vi "Main_15A.vi"() -> ()   [LabVIEW 2024]
uses:
  Utility/Universal Utility/TypeDefs_Utility/Cluster_Row-Column.ctl
  Utility/Universal Utility/TypeDefs_Utility/ENUM_4 Directions U-D-L-R.ctl
  b5234449-2328-4583-8824-3fa0b55a92a1.vi
  <vilib>/Utility/error.llb/Trim Whitespace.vi
  <vilib>/Utility/error.llb/Trim Whitespace One-Sided.vi
panel:
  out "Direction":T1
  out "Grid End":string[][](array[string])
  out "Array 2":T1[](array[typedef])
  out "Start Position":T2
  out "Grid Start":string[][](array[string])
  in  "Example 1":string="########\n#..O.O.#\n##@.O..#\n#...O..#\n#.#.O..#\n#...O..#\n#......#\n########\n\n<^^>>>vv<v>>v<<"
  in  "Use Puzzle":bool
  out "Answer 1436690":u32
  in  "Puzzle":string="##################################################\n#.......#....O....O......O..O#.OOOO....#.OO......#\n#..O.O..#O..#O..#O.OO......O....O..O....#O.......#\n#...O......O...O...O.......#O#.O.#OO.O........O.O#\n#..O..#O..#.O....OO..OO.....#.OO.....#.O#OOOOO.O.#\n#........O#.....O..OO......#.O..O#...O.O..O......#\n##O..O.O...#O.#...#O...#O..##......#............O#\n#.OO#O.O..O...O#..OO...#..###O....OO.#.O.##....#.#\n#.O...........O.....O..O.OO.O.O...O..OO....OO....#\n#OO..........O...O........O..##O.OOO.O..O..O..#.O#\n#.#O.....O.OO....#O..O...O.....O...........OO..#O#\n##.....O.......O.O.O....O.O...#O.O..O##....OO#...#\n#.OO......O.......O..#...O......#.OOOO.OOO...#O..#\n#.........O.O....OO..##.....OO...#....O.OO..OO...#\n#O....O..O..#...OOO...OOO#..OO......OO..O....OO.O#\n#....O.........O....#.#.O..OO......O.O..#O.O#OO..#\n#...O.OOO.O.O..O.........O.OO....OO.O.....OO..OOO#\n#..O.........#...OO.O#.O....OOO......O..........O#\n#........O.O.O.O..OOOOO.#.O.OO#OO.....#...O.O.#O.#\n#OO...O.#O.OOO....O....O.#.O.OOO.O..O......OOOO.O#\n#...#OO.O..O...O.OOO.....O.O.OO.#..O#...O..OO....#\n#O.OOOO.O........#O.##......#....#...OO..O.O.OO..#\n#.OOO.O.O#OO...O.O...O.........O........O..O#OOO.#\n#.#..O........#......O......O.....O....O.#..O....#\n#...#.....O.O.OOO.OO.O.O@O.O.O.O..#O....#.#.OO..O#\n#O.......#O...#O....O.#.....OO.#O.O..O.O......O..#\n#......O...OO.OO..O#....OOO.#.#....O.O....OO....O#\n#...O.O.#..OO#.O.OO...O.#.#..#O..#...##..O.......#\n##O...O..OO.O..O.OOO..O.........O#O...#..#.O..O#O#\n#O.O....#OO..OOO.#O..#O..O.#...#.#..O....O.O....##\n#.O.OOO.O....O...#O.O...OOO..O.....O.O..O.O..O..O#\n#......O...O..OO.O........O..........O....#....OO#\n#.O..OO.O.OOO..OO...........O........O.O....OO.O##\n#.O.OO#....#.........#..O...OO...OO..OO..........#\n#...OO...OO..OO.O...O.....#...O.#.....OO.O.O.O#O.#\n#OO......#...OO......O..O.O...O...#.....O......OO#\n#O...O.....O...O.O.O....O##OO.O..#..O....O#OO...O#\n#.O.O#OO..##.#O...O#O..O.O#..O...OO...OOO.......##\n#...O.#.O.#......OO.......O.OO..#.OOOOO...OO..O.##\n#............O..O.....#O.##.O.O.#....O#.......O.O#\n#.O..##..O....#O.O..#....O...OOO#.#...#..O...O...#\n#.O.OOOO..#.........O.O#....O....OO.OO.....##OOO.#\n#..O#...OO..O...O#...#..OO.OO...#....O........O.O#\n#.O.O..O....O...O.O.OO#...OO..O.OO.O.O..O...O....#\n#.O#..OO...#.OO...........OO.....OO#O.#..O.O...#.#\n#..................O.......O...OO..O..O.O.O.O##..#\n#.##.#..OO.#..........O#...O.O.O...##..O......O.O#\n#OO.O........####.......O.......O......O...##....#\n#.O........O..O..#...O.OO...#....#.#.....OO...O.##\n##################################################\n\n<><v>^vv<^<v<>^>^^<^^>>^>><vv^>^>^<v<>>^^>>v^>^<v><v><v>>^<^<<^^>^>^<<v^<<^^v><<><v>v^>^^<v<<<>v<>^>^^^><v<><v^<><vv^v>^>^>><^<vv<^>^<^<<<<<^<^vv><v>^v^^><<>>v<v>vvv^<>v<>v><<<v^<^<^vv<^v<>v<<<<<>v<^<<<^<^v^<^>^>>vv>>^^<>^^<^v<^v<<vv<vvv^<^^<>v^^><^^^v^>^>^^<<<^<v<^<><v^<^v^<>>v><^^v^vv><vv>^v>>^vv>v><v<>>>^>>^v>v^^<vv^<v>vv<^<>^>>^v^v><^v^>>^>^<<<<<><v<v<vvv><><^^v^^^<>v<>vv>v^>>>^<>>^^^><v<^<>v<^>^<vvv^>^>vvv>>v<>v<>v<><><<^vv>^<^<<>^^<v<^^>v^v<v<>>^^><>^>>>^v^<>^^^<>><v><>v><>v>^<>vvv>>><><v<><>v^vv^>v^^>>v<^<^<v^>>>^^>>v<<<v^vvvv>^^v>^v<^>^vv^v^v<^^>v>^vv<<v^^^v^<v<^v^<v><v>^^v<^^><^^<^vvv<v<<><>v^<>><<<^vv<^^<<>^^<^<^>^<><v><^>v>><><v^vv<<>>^^>vvv^><<^v<<^>^<^<<><^<>^<>vv>><v>^^<v<v>v^v^^<<>^>>^^v>>v>^^>^<><^>v<vvv>^>v<><vv<><^v>>^<^^<<<<<>^vv<<<v>^<><^<v>v^<v<v<v^<v^<>^v<vv^vv>v^^>v^>^^<v^<<v>^^v>v><<<<<^vv><v>>v><^^^v<^^vvv^^>^^^>vv<>v^<>><><<><^>^^^v^<v>>>v<>vv>vvvv^>>v<<<^vv>>>^v^v><<^vvv^<<>v<><^v><>^v>>v>^^<<>v^vvv><^^<>>^<<<<>>^>>v^^<>>>>vv>v<v^>^<^v>v>>^^>v^^v<^vv><^<^^<vv\n<<^<><v<^vvv<<vv<vv<><v^v><>><<v^<>^>>^>>^^^<^^v<vvv^v>v<>^>><^v>^^vvv^<>>>v>>vvv><^^v>vvv<vv<><v>>vv^^<>^^<^>v^<v>vv^<><v<^<>^vv>^^><>^>^v^<vvv><>^>><^<^>v>v>><v<<vv^^^>^v^vvv>>vv^^<^^<>>v<<vvv^<^<^>>v>>v<<v^<^v><v^><^>v^<v<vvvvv>>>^^v><<^^>v><<<^^<<<^><^<<^v<>^<>v<<<v>v<v<<<^v^^^<v<^^^<^<vv<>>^<^<>v^>>v^v><^vvv>^>>v><<^<<v>v>v>^v<v^<v^^v>^>>^<v^v<>^v><<>>>>>^>^<v<v>>^^v<><><<v>vv><^<>><v>>>v^v<>^><v^v^><<v<^^<vvv<v>^>vvv<>^>>v>^v<^^^v>v>v<>>^<><^<^<<v^<^>vv^v^>v^^^^^v^v><>v<><<<v^vv^>v<v<><>>^^<^<v<>^><>v^^>^^><>v>v^^>v<>>^>^^<v<^^^<<^^>^^>vv<^<^><>^^^v^^^>>^>>v<<^v^^v^<^^^v<^^>>^>^<v<>>^^>><vvv>v<v<>^<vv<v^v>^<v>v>v<>v<v<<<><<<^>>>^>^v>vv>>v^vv^<vv>><<>>v^>^^>>^v>^^v^v^<^<v><><v>v><^^^>^><v>vv<><<^^^<v<^^vv<><v<v>vv^^><><^v^<^v>v<<v>>v<vvv<<^<<v<vvv>>vv<<^<vv><>>v><vv<<>v<vv^><><^v<^<><<>>v<>v^v^<v<><v>^>v>v^vv>v<<v^>>><<<v<^v<v^^v^^>v^v>vvv>v<^v<^<<^>v>><<<v<>>vv>v><vvvvv>vv>v^<^^^<v<v^v<<v^v<^^>>v<vvv<>v>>^<v>^<v^<>^^>>^>vv^<>v^v^<vv^<>>v^^^v^^^^>^v><v<>^>v<v><>>><><^v><^^v<>v^v^>\nvv^^>v^^v<v<vvv<v<<v^>vv<>>>^v^>v>^><>v^><><v^^<^>v><vv>>><v<>v<<<^v<<>^^<vvvv^^>v>v<^>v^^<<vv^v>v^><><><<vvv>v>vv^<<<vv^<v<^>v^<^>vv<>>>vv>^^^^>vv>v^^v<>^^^>v><>>v<>v>>v<^<<>^>><^v<<^<^>><>vv>^><>^^^^^^>^<^<v<<^<<v<v^v>^vvv^<>^v^>><<<^^>^^<v>v^v<^>>><^^<v^<vv><<vvv<<^>v^^>v>v<v^v>v<^v>>v^>^<<v><v>^>^<v<><^>><>>^><^<<^v><^<<>v>><>v<<v<><^v>><^<vv>>v^<><>>^^<<v>>>v^>^v>v>^<v<>><v>^<v<v^^^>^>^vv^<vv<<<>><>><^<v<<<v>>v>^>^>v<><><^v<>><>vvv>^><<^^^<vv<vv><>vv>v^>vv>v><><<^vv>^vvvv<<<<v<v^<>>v>v><v^><v<<v>>^v^^v>^v<<v^^>v>><v<<v<^v<v^^<<<v^^<<v^>^^^^^^<><^>v^><><v^<^^<>>v^<v^v^^^<v^>^^v>v<>^><v>^^><^>^>v>>^<>vv<v<^^v<^^>v^^<>^<^>>>^<^v<vvvv>^<v^>v<<^^^<v<>^v<<<>>^<<^vv>>vvv>v<<>><>^^><vv><<<^v>>><<<vv<v><<v>^v^vv<v>^>>v<<v>v>>><v>><^^v^v^v<<>^>v^>><v^>>v><<vvv^<^vv^v>>^^>v^v<<<>^>v^^v<<vv>v^>v<<^^<<>>v<<v<v^>>^><>^vv^><^>v<<v><<<v<^vvv^v^^v^>><v>vv<>^>v^<<v><><v<^v>v>vv^^v^^<<>>^<v><>v^>>>v<^<vvv<<v<>v>v<v>vvvv>^v>v>^^>v>^><v<^>v><<>><v^vvv<^^v>v^^^^>^<v<>>^>v^<^<>^^>>><v^v>>^><^v^vv>^<v>v<\nv<^^vv><>><<^v^<^v^>^^<^>vv<<^vvvvvv^<><<vv>^<^v>>>><^v<<^<>><>><>>>><<^>>v>>^>^^>^><^<<v^v>v^v>^<^v^<>vv^v>><>vv>><>^<<v><v^v>v>>^^^<<^v><v<v^^>>^vv^>^^>^^v^<<<^>^>^><>v<<<v^>^^^>v<>^<v^v<>>><<<v<>^>v<^^<>^^v<^v>>^>><v<v>>^><^v<^<><>v>v>>>^<<><^^^<<<vvv<^>>^><^><v^<v<v><^v^v<<<><v<vv><<^v<v<<v^^<^<^^^>v^^>v><>^v^><^>>>v>><^v^v>v^<<>v^v<<^<<vv^^<v^^v<>^>^>^<>v>^v<>v>>v>vv^vv>^><><v<^<><<<>>><<>^>^<v<>>>^^<>>^>v^><^vv><^<^>>v>vv<^<v<><^v<^>>><^v<^><v><v^v^<<^><^<><^^<^v^^v>vv^^<v<<>^>>^^v^^<vv<<^vv<vv^<>vv>^>^<v^><><<><<><^v>^^v^><<<v<^<vvv>^><<>>><<v><>vv^^>>^^><<v><^<v>vv^^<^<^^^>^<v<>^v^>v^^v^<>v^<v^v<v><^>v^^><<<>^^^<<v^v<<<<>>v<v^^v^vv^vv^v>v>>^>>^vv^v^<<^vv^<v^v^<>^<^<v>v^<<v<<>^^>><v^>v^^>v^>>>v><<>><v^^^<><><v<<v<<^v>v^>><v<>^vv>^><v<^v>^<>v<<><>>v^v^>^>v>><^<^^><v><^>vv>v<vv^><^^v>^^>v^v<>v<v^^^<<><v>^^vv>v<^>vv^^v^v>>^vv^<><^<^<<<v<>><>>^>^^^^><^v<<<>v^<^^vv><^v>v^vvv><>v>^<<^^^v^^<>>v<^^v<^^^>>^vv<v^^<vvv<^<<^>v^<>^^^<^v^^<v>^><^>^^^v^^>^<>>^v^>vv<v>^<vv^^><^v^^^>v<^v<<>v<^<v\n<^><vv^v^>>^<>>>v><^vv<v^<^vv<<>v^>v<v^^^^>vv^><<v>^^^v<v^<<v<v><^^v>^<v<<^>^^^>v>v<^^>v^v><<vvv^^^>vv^v>^<vvv<vv><<>>>v>v<vv<><<><^v>vv><<^^^vv<><^<<^>^><<>^<v>^>^v<<>>v^<^vvv<v^>>v<<^>^>v<<<^v<><><^^<>^<^<v><<vv<>>^<v^^><^^v<<><vv><^>^^>v^vv^^<>^vv>v^>v>^v>v>^>^>^>><>v<^v>><^<>^v<>vv<^v<^v^<>^<>^<^^v><v^<vv>v<^>>v>>v^v^<^vvv>><v<vvv><<^^<^v<^<vvvvvv<v^^^>^^vv^^v>>>>>^^>v^>^><^><>>^<>v^>v<<<^v><v<v^^vv^<^^v>^v^<vvvv^^<^<^<<<v^v^^<v<<v><^<v><vv<^^>v<vv<^<^v<^>^^^vv^<>^<v>^v^<><>><v>v^<<><^^^>>vv<v^^<v>>^<<>v<vv>^<<v<^<<vv^^<v<vvv>^vv<v^><vv<><v>>^^>v>^<>>^^<v<v<v^<vv>><<^><v<v^<<vv^^^<v><<^<v<<<v>^<vv^><<<^^v<^>vv<>>^>^v^<v>^^v>>v^>>v>vv><<v<<v>v^vv^>vvv^^v<>^>^v><vv>^><v>v^>^v^^><>v<^<v>^<<^vv>^v<<><vv>v^>vv<>>^>>>><<^v<v>^<><v<<<<>>^v>v><^v^^>^<<<v<v^^v^<>v><^>^>^^^v><<<^>v><^><<^vvv<vv^v>v^><<><^>^<<vv^>v><>v>v<>v<vv<>v<<^v>^>^v>^^v<>v>v<<v^v>>>vv>>v>>><^^^v^>>vvv^^vv><^v^<vv^><<^v<vvv<^^v<<vv<<v<><vvv<><<>v<v>^><<>><v<v<>^<v<>vv<<><<v^>^^^^^><<><^v^v<^>v<^^^><<<^<^v><^v<>^>>v^v^<^^\n>vvv^<<>vv>vv<^^vvv>vvvv^<^>v^<vv^^v>^v<<^<<v<<vv>^v^v<<><v<><<>>><><v><<>v<<>>v<<<^>><v<v<>>>>vv>>>>^v<>^><v>>^><v<>^v^v<>^v<^v>^v^^v^^v<><^v<<>^<>><v><^<^<<<><^v^vv<<<<>>>^vv<<><<v^^vv<>vv^>v<^v^>vv<>vv<<v^<>^<<<>^><v<vv><>^v>vv^><<^^<v<<v><>^>>v><>^>vv^^>>^^<^>^^<^vv^^<>><v<<^><<v^^^<v^v<<>>>>^v^<v^>>^><<v^<v^^>>v<<<v>>>^<v^^>v^v<>^>>>>>^^^>v>v>>vv<v^^>>^v>v^^vv<<vvv<<>^^v<<>>>^<><<<>v<>>^v^><<>^>v<>^^^>v>vv<vv>^<^^v<^^>v<^^^^<<<v>><<vv<v>v^>>><v^v>v^^^v<<<v^><>><^<^<^>><>^^v>v>v>>v<>>>v^^><^v<^>><v><v^<^<^>^^^>>>v^<>^>^v^v<vvv<^^^<>><<v<<>><^v>v^v<>>vvv<vv<<><v<>^<<^vv<^vv><>v<^v><^<>>>^<v<vvv<^vv<^vv><^v^><<<v^^<<^v^v>^>v^^^^v<>^^^<<><<vv<<^>vvvv^vv>^<vv<^^<^>^<^^^>v>v^<<>^>^<<v><>^v^^^><<><>v><<<><>v^>v>^<<<>v^>^<<^vv>>>^vvv<>>vv<vvv^<v<>>>v^vvv^v>^>>v<v^>><v^<^<^<^v<vv>v>^><><><^v>>v<^^^v>^vvv^^>>^<^<^^><<>^^<v<<^>^>^>v><>v<<v><<>><^v<>v>^<>^v^>v>^<>^>^>v^<v^><<>><<>v<^v>^<<<<<<v><<>><>><>><^v^^^vv<v^v<vv>v>vv<v^^^v^><v^^v<>v><<>v>>><<v><^<><>^v<v<><<<><>>^<v^<v<v<v^v<v<><v^<>vv\n<<<v^>v>>^>v>v<v<>^^><<^^><^^vvv>>>^>^><<^^<v<><v<<>^^^^vv<^<v^><<v>>><<<<<<<vv<<><v<<<>v<v<<^vv^<v>^^^^^^><^vvv<>v^>^^vv<vv><^>><v<>><>^<<vv^^<>^>^><v><v>v<^v<v<^^^^><^<^^><^v^^<vv^<><<^>^v<v^^v^^<>><<v<^^^<>vv<^^vv^><v><<v^v>>vv^><v<^^^v<<v<<<>vv>>><v<vv>^<^<v<v<>^>v><^>v>v<^<>v^^>>^^<>^<^<v>><<^<<^^^v<v<^<^<<v<v>>^<>><^v^v^<>vv>><v^^><v>><^<^>>^^<<v^<<<>v<^<v^v<v><<^v<vv<v<<>^v^v<<><v^><>><^v^vv^>>v^^v^^^<v><<<v>>^v^><^<v<<>>>^v>^^v<><vv<^^<>^^<<v<<v<<v^^^<^v^<<>vv><<<vv^^<^^vv<^v>^<v>^^^vv^<>v<<>^vv<<vv^^<>v<><^^<vv<<v^<<^<^vv>><^>><>><v^<<v><>^<<^vvv^>v^^>v>v^^^^^^^^v^^^v^<^^^v^^vv^>>v>v^^<v><><<^>v>><^>^v^><^^v>v^vv<v^>^>^<<^^^vvvv<<>><>v<>vv<vvv<<v^^v^^vv><<>^<^>^^^^^vv>^><^^^<<><>^^v^>^^>>v^^^<^<><>^<<>>v^<v<^v<>>>^<vv>^v^>^<<>^v<<v><^v^>><>^<><<v<>><v<>^>^vvv^^>v^>>v>>^>vvvvvv>>v>^vvvv>>^^^<<v>^^^<vvv<<v<v^v^^v<><<<v^v<><<vv<<<<vvv^^^<^>v^v^v^^>^v>^<>^v>>><^vv>vv<^^^vv<>^<><><>vv^v>v>v>>>^v^<^<>^<v<v<v><^<<>^^<^<>^v>>^v^>v^>v^>v<v^>^<>v^<^<^<vvv<v<vv^v<<>>^<^v<^^^<<<^>^^>^<<v>\n^v<v^<^^>>^v><v<><^<><><>v^<>^><>v<<vvv<><>v<><<^^vv>>^^^><^^<>^>><<^^>v><v><^>^>^>><>v^<><><^^^v<^<v^<>v>vv>v>^<><<><^^<^^v<><^<<v^<<^>^^>>>^>>^^^^<^v><><<<^^<^v>v^<^v^><v>^^^><^>^vvv>^v<>v<v><<<^v>^<v<<>^^^<^>^^^<^<v<<>>>>v^>^v^>v^v<v<<^<^^<v^^>v<><^<><^>v^v><<v<v>^vv<^vv><v<v<^><>^v^<<^>vv<^^v<^vv<>>v>>^<>^>>^>>>>^v^<>><v^>vv^^>^v^>^<<<v>^><<>>>><<>^v<<>>>>>^>^^^>>><^>>v^vv^^v><vv>^v^vv^vvv^>^>v>v^vv>^v^^<vvv>vv>><<<<^<<<><>v^v^^^<>^v^<>><<^^^<>vv<<<v>v<<<^>><>^<><v<v>v<v<vv^vv<v^vv^^<<<<vv<>vv^vv<v<<v<v><><>^^><^>^<><^v^>>^<^>>>vv^><<><<^>><v<<v^v<>^v^^v^<><v>^v^^vvv<<v^v<<^^^^^<vvv<><^<>^v<<>><v^v^>>>v^^<^>v<><vv><<<<^<v<v<<<^>v<<<v^v<<^v>^^><<<v>vv<<>v<>v^v<^<>^>>><^v><>^^v><<>vv^v<^v><vvv<<vv<><^>>>v<v><<^^<v>^vv^^>^v<<^<>v^v<v><<>^vv><<<vv^v<>^<v^v<^v>^<<<>^>^vv^><>v^<>v<>>>^vv<vv^<^v^<v><>>v><vv<v>><^v^^^^>>v^>^>v^^<<^^v>vvvvv<>^vv^<^<>^<>v>>vv>v>v<>^><>v^^^vv^>v^<>^vvv<>>>v<<vv<<v>>v>><<^vvv^>v^<<v<v<<>^<><^v<<^>>>v^<^>v<<<<v>^^^^^v><>v>vv<>>^<v^^^v<>v<<>v^<>>v><^^^v^^^>^^>v>\n<>^^<<vvvvv^>vv>>>^<>^v^vv<v^<^v>^^><^>><<^^vv>v<v><v^<^<^>><><<<>v^v>vv<v^v^v>><><v>>^<v^<><v<^^^v<v<<v<<^>^v<^^>^^^vv^><>>^<<<<v<^^<v^<<^^<v>>v^^vvvv^vv>v>>vv<^^>v^vv<>v<v<v<^<v>v^>v^>>^<v><<<<<^^<>>^v^<<v^><v><>vv<v>^^<^<><v<^v<^^vv^<><v>^<<^<>^^^^^>^vv>v>^>>vv>v<>v^^<><^^>^>><>^^v>v><v<^<<<^v<>^>^v^^v>v>>^>^vv><^>^>^<><^^v><v<^>v>vv^v>^v^>^>^v<v>>v>>v^<<v^>v^>v^>>v<^<<<><>^vv<>>v<^^^>v><<<><<<vvv<v<>v<^vv^v<v><^^vvv>^^vv^<>>v>^vv^^<^<>><<>v^v^^^^^<v>v^^<<^^<^v>>>^>^^^^v>^^v><^v^>^v>^^^<>^<<^v^v>v><^^v>^vvv<<>>^v^^>^>^v<v^>>>^v><v<>vv^v>v>v^v<^v>vv>>^>v^<^^^^>^<^>v^^>>^<>^^><v>vv<^>^^<^><<>>^>^v>>v>^<^v<<vvvv^vv<>>v<><^v^v>^v^^v^v<v><<^^v><^>^>^v<vv^^^^<^^v^v<v>^><<<v><<<>^v^>v>vv<^<><^^<>^<>>vv<v<<>^><^^^^v>v<>>v<<>vv^>^vv><<vvv><>v><^v^><vvv>vv<v^<>>^v^^<<<<>>><v<>>^^><^><v<^^<<<<^^^>vv^>^v<<v<vvvv<>^^v>^>v^^><<^<^v><v>^^^>v^<>>^>vv>><^^><^^^>^>><^<>>>>vv><><^<>>v<>v>^v^>^>^><v^^>v>>>^v^vv>v>><>v^^^>><v><>v<>v^^^vv<<vv<vv><><<^<<<>vv<vv>v>^^<v>>v^>>v><<v>^^<><>^>v^<>^vvv>^<^v<<vv<\nv><^^>v>v>^<^<^<<v^<<v><^^<<<^^>><<<^>^^vv<^>vvv<>^^^<<>^vv^v>^^v>^v^^v^<>^vvvv^>vvv>^^<<v>v>^>vvv>><<<v>>v^><>>^<<v^<^^v>><<^^^^><v^<<^^>^^v>^vv^>vvv>v^v^vv^>>^<^<>>v<v^v><<^^^><^^vv^v>v>^>v<v>^><>^<>^>^>vvv>>^<^>^vv>^^<>^^>^><^>^<v<>>^vvv<vv^v>>><<<v^>^v^><^v^<v>vv<<<><<<vv^^vv>>v<v<>v<><^^vv<>>>^v^^<^<<>^<<^<vv^<v>>>v^<>^>>vv>>>^^v^v<vv<^v>v<<^v<^<v^v>v<v>^^><>v^v><<<<v<>>>v^vv<^>>^><v>^v>^<vv<<^>^>v^^<^^^^vv>><v^^v^>^>><^v<^v<>v^>v<<^<v<vv<<^<>vv<>^<v<>^^vv<^^^^<^>^^v>v>v>v<vv>v>v>vv^^<^^<vvvv>v^<^>vv>>>^^^>>>><^^<^<v>v^^v>>>>>v>^>>vv<v^>vv<<<><>v>vv>^><<>>v^<vv<v^v>^v^>>^v^<>^v<^v^<v<^v><^^>v<v<>>><>><^>>^v<>>><><<v>^>^<v><^<^<<v^>v>vv>>vvvv<^>^><>v^<>^><<v^^^^^v>^>v<v^v<>>>^^vv>v>><^^<>><<v>vv<<<>><^v><v>^^<vvv^^^^^<^v>^<<v>>^^vv><<<v<>v^<<><v<>><^<>v<<^v><vv>>^^^v>v><^^<v^><^<v>vv<v^^^^^>><>^^<<>^>>v^^>v^<><>^v<^v>>v^vv<>v<<^<v^v>>^>><v<^^vv<^^<^<v<><^vvvv^>v^<<<><<v>^^^><^><v>^<<^^vv^vv>v>v<^>>>>^v<^v>^v<<^>>>^<<^<v^^v<^<v^<v>^^^vv>^<>^<^<^><vv>>>^<>^^<<<<<v^^>>>vv<^^>>>v^<vv<^\n>>^>^^>vvv<<^^vv^<^>v>^<^<^<^>v^<v>>v>>v>^^>^<<>>vv>>^>>>>>v^<v>><v<>^<vv<>>><v<^^^v<v^<v^>^>>>v>^v^v<^v<>^^v^^^>>>^>v<^>^<<><v<<<<v>v>^<^^^<<>^<v^>>^<<<^>>^>^^>^v^^><vv^<v<v^v^<^>^<v^vv>^><^^^><^v<<>v<^<^<v>^^>v>^v><>^<>v^v^<^<v><>vv<>vvvv<<<^v>v>v^^<<vv<<<<v>>v^^^v>>v><^^^><v<<^v^v>^<<>>><^^v>>^v>><><><<vvv<^^>^vv<^^v<>^vvv><<^^<v>>>^>vvvv^^vv<^v<v<><<vv><><>>>><><v>v^><^vvv>v<<>^^^v>><vv<v<^<v^^<<>><<^<><vv<>^><>>><^v>^<>>vv>><>^>^<>v>v<v>v^^>^^^>^><>><>v<<v<<<<v<<<^v<<<<<^>^v>^v<<<>v>><<><v<<^<>v^v^^v^^<^>>^^^^v^<<<v<>^^<^>>>>^^vvv<><^v<<^^>v>v>^v><v^<^>^^^^><<>^>^v<^v^><<<>^<^v<<v>^<^^^>^^^^^<^^<v<>vv>^<^<<vv<^^>v^vvv<^<vv<^><^^>^^v<^v<><><>>v><v^<><^vvv^v^vv^^<^<^<<><^<^<>>^<<<^^>v><<v^>^v<>>>>^v<^>^^^^v>>^v<^>>v><^^^<<^<<v^>vv>v<^^vvv^v>><<>^><<^v<v><v<><vvvv^>v>>v<^>^>>^<^v^>^v^v<<^<^>^vvv^>>v>^>v^vv>>><<<vvv<v>^><^>vvv<^v<v<<v<v^v^>>^vv^><v>^v>v>v^v<^<v>^vv>v<v>v>>>^^<vvv>>><<>^<>>^<v>>^^^<^^v^v><>>>v^^^vv>>^<^v^>>^v>>^<>vv^vv>^^><v>v><>^><<>^<>^^^<><^><v<<<<>>>v<<<v^^^v^^v>^<\n>^^<<>v^><v>>^v^^<v<^<>^>^v<><>^><<>^^>>^^>><>>vv<^v<^<>^^v^v^v^^<>v<<><^vv^>vvv<vvv<v>v^v^<<vv<v><^^>>v<v>v>^vv>^^^v<v<>><v^>>v<^<v>v^v>vv><>v<>>><v^^<v<<v>><^>>><v>>v^>^v>v^^v<>vv^><^v^>^^^vv<v^>v<v>^^v^>>^v<>>><v<^>>v^<<^>>>^<^>>vvv><>^<v<v<^>^^<^<>>^^v><>>><>vvv>^<<v>><>>^>><^<v><^><>^^^<^v><^^<<<<^<<^v<><vv^><^^^>^<^<<><vv^>v^<^>><>>^><^<>^>v><>>v>>>vv>^vv^>^^><v^^v^<<>v^^^vv>v>v^>>v^<<<^vvv><><><vv<><>^v>v^<>>>>^>><v<^^^vv^^<>v>v<^v<<v^<^vvv<<><<^v>vvv^^v^^><^<^^<<v^^<<^<^<<<>v<v<><>v^>vvv^<^^^v^v^v^<><v>vv>>v>vvvv^>>^v<^>>^v^^^^><^<v<^^<><^^<<<><>vv<<>^^vvv><vv^v<v<>vv<<>v<v<v^v>v>><^v<<^>^>>^v^<^vv><^>v<^v><v>^^v>><^>^>^^vv^>^v^^^v<v<<<<<v^>v><>><^v^vv>>^>><^><>v<<>v<<<v>v^^<<^>v<^><^^^><<^<vv<vv<<>^>vv>v><^><<^<>>v><<<^v^^<<<vv<>^><<>v^v>vv<<v^v>>v<<v^^vvv^<>><^v^<v<^^^^>>>>vvv>v^>v>^v>v><^^^<v^^>>>v<v>^>^^>v>vv<>>v^^v^>vv><<>v^>^^v<<>vv^^^><<^<>v<vvvvv^^^>^vv><<v<^>v><><><<v^>^>^v<vvv>v><v>><<>><<^<^<v>>v<v<^<><<v^>>>^>><^^^>^^<><v>^^<^<<<v<^<v>v>>v<v>>^^v^>v>>^v>^^>><<>v^><>\n^<v^>^>v<<^^<<<vvvv<^v<v^^^><vvvv^^<>^>v>vv<v>^<<><><^^^v^<^>^>>^^<^>v>vv><^^>vv<>^v<v>^v<^v>^>><<>^<v><v^>v<>^^vv>>^vv>^v^^v^^^>>>^<<>v><><<^<><^^^vv<v>v^>>^><>^^^<<^^v<^vv<<>>>^v<>v>v^<v<>^v>vvvv><<<^v>^>v<vvv<>>>^<>^<v^>^<<^v>^><^<^<vvv>^^>v<v<v<>^vv>^>>>^v^<>^<vv<>v>v^><v<^^<><v<>><vvvv^<<^<^<^v<^<^>^v<><^<^<>^<v<v^<^><v^>^v^vv>>^<>v^<>^<v>v>>v>><>v<>>^<v>>v<vv<v<v><>^<>^^>^vv^v^<v>>^^^v^>vv^^>^^^<<^vv>^<v>vv<^v>^v<^><>>^v<v<>v<v>^v^<v>v>>v^v^>>^^^>^v<^v>^^v>><^v^<>^<v<<v^^v^^><^^v<><<>^v>^>vv>^<>><v>><<<>v>^v^>v>^><<>v<v^^v><^v>^^<^>^^v<vv><vv><><^<>^><^<>>^^<<>^v^^>^>^v<^^><v><^^^<<^><<v^<^v<<v>vvvv>^^v<v^v<<>v<<>^v>>vv>>v><>^^<v>v>v>>^^>^<vv<^v>^>v<<^>^vv<<<v<vv<^>v>v>^^<v<vv>^><^>^v><v<<^v^v^>^<<^^v<<v>^v^>>><^>>^<^v<^v^>^v<>v<^v^<^^><><<^^vvv<^><^^<v>v><v>>v<^>vv^v><^^^v^<>>vvv^v<^<<>v><><v^>^><<>^<v<<v^<v^^<^<><^vvv>^^>v^vv^>vv<v<<>^><<<<v>>v^<>>v^>^><vv^v^<^><^vv<^>>vvv><v^>v^<><^>^^v<^>^>^^<<^<<>><^v^>>><^v<v^^^^v<><>>^v^^v<<v<^<vv>>>v^>^v<<<>^v<<><v>>v<<<vvv>v>><^>><vvvv^^\n>^^v<v^<v^<<v<v>^<<<^^><<>v^<^^<>v>^>vv>v>v^>^v^>v<>v<vvv^v>>v>vv<v>vv^>^><^^vvv<v<<><>^<<>>^^^v>>vv^vvv^<<v^v<v<^<<<<<<v>>>>^^^>>>>>>^v^><<v^<v<>^<v<v>>>^><<<v><^^<>>v^<^>^<>v^<^>^>^v^><^<^vvv>v<^v<>vv^^^>v<v>vvv<^<v<v^<<<>^<v<<^^<>^^>v^<vvv^<v^v>><<v>>^v>v>vv<><>>v<^v^><<v<v<^v<v<<><^<^>^<v<>>vv>v>^>v>^<v^v<^<^<<>vv<v^v^^v<>^^><>^<>vvv>>^^^>v>vvv<<><^v>>>^v^<v<><^^^vv>^^v>v>>v><v<^^^>v<<>^><^v<v<v^vv<><>v><<<<^v^>>^v>vv<>v^<vv^v^<^^>vv><^v^^<v<><v^<><^<<>v<<><<>>>^><<<v>^<^<v>v^^<<>>>><<<<<^>^v^v^>>><><>>>>>vv<<>^<v>v^vv><<^^<><^^<^^><<vv^<^v^^vv>>>>v>vv><>v>vv>v>vvv^<v<<^v<>v<<v><<v><><^^^^^>^^>><^v<^^<vv<<<<^v><<^v^<>>^^v<v^vv<><<vv<v<^<v<<><v^v>v><>><>v<^<v<>>>^><>>^^v>>>v>v<<><^<<vv^^><v<v>>vv><<>><<^>v^^v^>>>^v^<>vv<vv<vv<^^><<vvv^>^><^^v>^><>^<<<v^>^<v<<vv><v<^v<<v<>>><<><><<<vv>>v>>><>^v<<<^<^<^^^<<vvv^^>v<v^v<<^<><<v<^>><v<<v<^^v^v<>><<<>>^^^<v>>^<v<>^^>v^^^^<>vvv^<^<<<^^^>^<>vv^<>^^^^^<v^v>><<^<^^<^^vvv>v><<>>v^<<<>^^^><v>^>>v>^^><v<>^v>v<^^>v<^<>^^^<>^<>>v>^v><>v^<^>^>vv<v^\n><<^v<>v^v>v>^^>v^v<<^<<v^^>v<v<^>>^<v<^<>><vv>><<<^^v><v<><^>^<<>^>v^v>>>v<v>>v>^v>>v>v^<^<>^vv^><v<^v<v^<^v^<>v^v^v^>>^><><<v>^^<><^<v^>>^<>^<v<<<>>>><<>>v^<^<^<v>^><^v^v^<<^>>^^<v>^^<>v^v><>><<v<v<>^>><>>vvv<v>^<<v>^^<>^v<<^<<^^vv<^v<^>^<>><^v>>vv>v<<>><<>>^><vv^><>v<v^v^^v^>>^v^v>^^<^^<^^^<<vvv><>^^^<^<<<<vv<><v><^vv<>vv>^^>>^<^^v^>^vvv^^<v>^><>>^<<>>>><><v<^<>^>v>^<>v^v<<v>>^^v<^><^<^v><<>>>><><v^<><>>^<vv>>><vv>v<vvv>v^<^vvvvv^v>><<<v^>^>v<<<>^v^^vv<>^vv>^<v><^><><^>vvvvvv>v<^<>>v<><v^><^<>vv>>^^v>>vv<v^>v^v>^^><^^>><<<>>><v>>^v>v><v<^<>>^<^vv><^v<<v<^<^<vv><vv<>^^^>^>>>v>^>v<<><^^<<>>>^>><<v<v<<<^^>v><^>v^<<v^<>><<^<^<>>v^vvv<^^v><^<^v<>^v>v^><>vv<v<v<^v>^^>vv^^>^<v><^<^<><v<v><>>>v^>><<<^<^>vv<^^^>><<<v>^>v<>v^^>vvvv^<<<<>v<><v^>>^>>v^^^<v><vv>v<>>vv<^<^><v<^^<v>v<<v><^>vv>^v^>v>v<^<<><>>^v<<>v>^v^>^<v><<>v>^^<><><v><>>v<<v^<v<^><>^vv<><>v^<vv^^^>v<<vv>>>>>v^<>>^><>>v<<>v<vv^v><>vv<<vv^v<>>^^<v<^v<v>vv>^>>v>vv^v>v<>><>>v^v>>^>v<v^>>>^<v<^^>>v<<<vv<<>v><<><^v<>>vvvvv^v><<>^v<v>^\nv>^>v<^v>v><^>vvvv<<v<>^^<<>vvvvvv<v<>^>>><v><v^<<^>^v<>v^>^<<v<><vv>^v^>>^<<v<v^>^>v<><v>^>^^v<^>v<>^><v^>v<v>v^^>^^<>^<<^<<<v>>v^<^>^>><v>>^>>v^<^vv^^^vv>v>v<v>v^>v>^><<^<><<<<>v<vvvvvv<><v>^<>^>>vv<<^vv>^>^^>^v>vvv^vv>>v<^^>^^>v^<<vv^>>vvv^vv>vv><>v^v<^><<>^^vv<<^vv><>^<>>^^^vv^v^>^>^<<vv>><^>>v^vv>^><v<<vv^v>>v<^<>v<v><v<><^^vv^^<^<v^v>>^<vv^<<v^<v^^^><<^>^<<^^^>>vv>^>><><^v^>vv<>^<vv>>v>^<<>><<v>^>>vv<>^>>>v<vv<v^>>>>^v^v^>v^<^v<<>v<<<v<^<>v><<^v^<<v^<vv<^v<><^<^>v^<v>^vv>>v<v><<<^v<v<v^^>>^>v^v^>><<>>vv>>>>v^v<<v^v>^>v<vv<v<<>v><<^<<>vv>^<^>v<vv^^>^^>^<^v<>^<^<v<v^^v<^>>^<><^<<>^>^v^v><<>vv^v<v><>^^v>>^v><<v^^^>^v<><^<^^^^<>><<^^<<<^<^<^v<>^<^<v>vv>><<vv^>vv<>>><^^><^vv>>^v^<<>>>v^^^<>>^^>>vv^<vv^>v>>v<>v><><v>vv>v<<v^<><<<v^v><v^^v<<vvv>^^<^v<>^><v>>>^^v^<^<>^^v<^<>>>><v^>^^^>^v>><v>>v>^>^v>><>v<v<v<>v<^^><<><>^v<<<><>vv><>v><<<>>>>v><<^<^^>v<v^v<<v<^>><vv>^>v<v^v<<^v^^>v^<v^vv^vv><^<v<^v<^<>v<v^>v>^>^>v><^v^<><<v>>^v^><><<>^>^^>^<v^>v>^^vv>>v<v>^<v<v^v^>^>v^v<vv<v^^vv<<v<<^>v>^\n^<<>>>v^^vv<>^<>v>^v>>^vvv<><v^^^<<^^v<^v<^><<<><v>^<v^<^^<^v>^>vv^v^vv^>>vvv<vvv<^><>><><^<v<^^><^^v^v^><vv><<^vv<^v<v<^v<^v<<v>^^<<><>v<>>>^v^v<>>v><<<<>><vvv<^<<>>>^v^<<<^v^>>vv^v<^<<>^^v>>^^^^<^>v<^v^<><v^<<<^v^v^v>^>^>vv><<^vv>><>vv><v<>^v>^>>vv<^^<>v^^<^v^<^v^^>v>>^<v<<>>>v>><v>^^v^>^<>><<>>v>v^>>><>vvv><>>>v>^<<^v<^v<^<>^v<^>>^<^^><^^v<^<^<>vv<<v<^^v^<<<>v<><>vv^v>^>v^<v>^^>v<<v^>>>>v<^<<v<>vv<v<^^>>v<^v^^^>^<><>^v<<^><<v>^<v^v^<^>^>vv<v^^^^v^^^v^<>><^>>v<^v>v<>>>^<^<^<v^>>^<<<v<<v^^<>^<v>>v>^<^^v<v>^>^vv>v^>v>>vv<<><v>^v>^v<<<<>^<<<<>v<vvv>>>>><<vv><>v<v^<><^v<>v^^<v^>^^<<><^><<^v<<^>^<v^<^v<^vvv<^^<v<>v^v<><<<v<>>><v<<v^><<^^>^<>>>v^<>>v>><>v><v^><^<>>v^<>v^<^>v^<^<<>v<<<vv>^>>v^<v^>^>v^^<<^>>^<^^>><v>><v<<v<<>^^^vv>vv<<>^<v^><v<>^v>^^^^>v>^^<<^<^<^<<v><vv^^^v^<>v>>vv^><<>^^^<^>>>vv<>>v>^<>^^^v<^vvvvvv^<^^>><^<^v^vv<<v<<<>^vv><>>^v<v^^><<v><v^>^v^v<^v>>v^v><^>vvv<<^^<v>^^<<v^v>><<<>v<^>>^v<v^<^vv^v>v>v<v<vv^^<^<>>vv<v<v^<>v>^>v><^^^^<>^>>v<>>^<v><^vvvv>vvv^>^v^<<v>^>>^<<^>vv<>\nvvvv^v^^^<<^>^^vv<<^>v>^v>^>^>^^^^^^>v>>vv^>>^^>^vv<vv^<v<<<^<^<<<<^<<v^^^v^<<><<>^>^>v^<vv<vv>^>>^^v<v<v>^^v^^^^v^<<>^<>v<>>^><><v>^<vv><v^<vv<v^>>^v^^vv^>^v><<^><^^vvv>^^><>>^v>^^>v><>>^<>><^<^>vvv<>v^<><><^v>><^>^>^^^v>><>^>><>^<vv<v>^<v><>^>^vv<vv^^^<^<v^^v>>^>><v^^<>vv>v^vv<vv<v<<<^v>^<v>v^<<^<>vvv^v<<v<<vv>>vv<v<v<>v^>>><><v><^v<<^><vv<^^>^vv>>v<>vv>v^vv>^<^v<<><<^>^>vv<v^<v<<><>^>^><v^^<<>^^><>v<><^^^><v><vv<^^vv><v<^<v<^vv^<<^>vv>^>>>v^v>v^>^>v^vv>>><v<v<<v^>>v^^^<>^>^>v>>^^^>>>><><^<>>^vvvv<vvv^^vvv^<vv>>>>^v^>vvv<vv>^><^><v><<v<^v><v^<v<<>>><<v<v<<^>^v^<v^^<>^v^<^^>><v^>^vv>^v<<v>>v>v<v^vv><<><<^><^<<>^<>>>^vv^^^>v<^^^v>^v<>v^^><vv<<^^>^^^v>v>v><<^^<>><><<<^><>v<^<<>><v<<vvv<<vvv^>v^vv<vv<>^^^<^<^><<vv>v^>>v<<v<v>>v<<v^<><v^^>^^<>^v<><vv^<^v<<<>^<<^^v>v<^vvvvv>v^<^><v<><<<^<v<<<v<vv<^^>^<v<v^>^>v^^v>>^vv^>v<<<v><>^v><v>v<>v>^v^v^<^>^>^^v>><v^v<v>><<>^^^^^<vv^v^^<^>>>v<<vv^><v^v^^>><>^>v^>v>^>v^>vv><v<^<^>^>^v^>v<>><<<>^v>>vv^v<<^v>>><<><<<>^<vvvv<v<^<<>vv<vv<v<><vv><<^^vv>^><\n<^^^<v><^<vv^^v^><><^v<^>v^<v<>^v^v>^^v>>v^^>^v<<<vv<^v^><vvv><^vvv>>><>><^>><>>v<>v<<<^^<>^^^^>>^<^v^^<v<><<<vv>v^^^>>^<><^<>>v>v^>^^>>^v^>^^^^>v<^><>^<>>v<^v^<<>v^v^<>^<<<>v>^>>v^^v>v^v>^>v^^>>>v<^^v^^>>v^>><^^<^<<vv>>v^<vv<<v<^^^v<<v<v<v<>^v><^>v^<^vv<>>^v<v>^>v>^>^>><vv<<><<vv^v>>^^v><^<^^<<^vv><vv><<^v<^^^^>>^><v<^v>>v>>^>^<><^vvv^^<v^^><^><^^v^<v<<^v<><^><><<^v<v<^<v>^>v<>vv>^^^vv^^^^^<>v<<>vv<>^vv<^<^>^^>^^<^v<<<>^<v^<v<>vv^<v>^v><^>^v^<<<^<>v<<^<vv^v<^v<v>>v^^v^^v^v><<v<vvv<^<<^vvv^^v>v<<v^>vv><<^<^<^>^>^<>><>v<><>><^^><<<v<>><v>^<<<<^<<^^^^v>><^^v<v><v^v<^v^v>^>>>>v<>v<v^v<vv>^^<v^^^<v^v^<<^>v^><>>>v<>^v>v^^>><>v>^v^<^^v^v^^^v>^><<^v^vv<>>>^<<<>^^<>^^^vv^<v^>v<<<v>v<>>><v^><<^>v^^^v>^<v<^<>^^>vv^>>><><<^<v^^vv^>v><vv^^v<^^><<v>v^>>v<v^^^<vvv^^<<<^><<^>><>^^v<^^v<^^>^<<>^vv^v^^<><>v>v^^^<^^<v>><>v^^vv>>^vv^^>><>v^vv>vvvv^^vv^><v^^^>vv>^vv<v^^^^^v>^^><v^<^vv<>>>v<>>>^^>><<>v<^vv<<><v><>v><v^<<<<><>^^vv^^<^v<^>>>>vv<<^<>v<^<><^v^<<v<<>^<<<>^>><^v<vv>v>><^^>>^>^<>^^>>v<>^<<^v<><v^\n^<>vv<vv^^>^<^<vv><>>^<^^>^>^<^^v^>><>v^>v>v>vv><^>^>^>><<>^><vv>vvvvvv<<v>^^<<<><<^v<<^^^<>v<<<<vv^^v<><>^v^^v^>^^><vv><^vvv^^<^v^><>v>v<>v<<v^>>^v^>^^^^>>^v<vv>>><>^<^vv^^<v^vv^^^>^>^v^>>^^>>v><>><v^<>>vv^>^>v>v^<>v<<^<<^>v<<v<>v>vv^>^>v^<v<>^<>^v<>><vv<>><<>vv^^>^>^^v^^>v>^<<^<><v>>^<>v><>^>>v^><^^v<vv^v<v^>v^^<v^>v><>v^^><<><<><>^^<^<>vvv>v>v<>v>^<<>>^v<^><<<vv^>^<<<>v<^v>><^^>>>^<^<>v^^^>>>>v^>^<><^<<^><^^^<>^^>^^^v><^^<^v<>><<>^v<><^<<^^>><<><<^>^<^^>^>^<<>>vv<<<>v<vv>^<>v^>><>v>^^^>^><<^^^>>^^v^^<<><^^vv<>v^<<v>v>^vv>>vv<v<v<v<>v^^<>><^<<v<><>^v>^>v>^^vv<>^v^^>>^<>^<<^><^^^v>^v><v^^<>v^^<^v<<<><><<vv<>^>vv>>^>^<>^>v<<v<<><>><^vvv>>><v^^<^vvvv^v<^><><<>v><><<>v><^^^v><^<^vv>>><^^<^v><^<^^<v><^^<v^vvv<vv>v<<>^^^v><<><<vv<^<<^v<v<v><>v^>^<<<<v^v>>>vv>v^^^<>>>^<v>v<v>^^>><v<>^vv><><<<>v><^><v<v<<<vv><<vv^<<>^v^v<<^<<>>^>^^vv^>>>v>^><^vv><v<vv>^>><<^>>>^>>^>^>>v^^v>^<v><v^<<<^v<^<<^<>v^<<^<<v<><><v>^^v^^v<<^>v^v^>v>v>v>><>><<v<v<<><^>v^<<<^>^^<<<>^v>><v>v<vv<><^><<^<v>^v<<v<^>^v^^>vv"
  in  "Example 2":string="##########\n#..O..O.O#\n#......O.#\n#.OO..O.O#\n#..O@..O.#\n#O#..O...#\n#O..O..O.#\n#.OO.O.OO#\n#....O...#\n##########\n\n<vv>^<v^>v>^vv^v>v<>v^v<v<^vv<<<^><<><>>v<vvv<>^v^>^<<<><<v<<<v^vv^v>^\nvvv<<^>^v^^><<>>><>^<<><^vv^^<>vvv<>><^^v>^>vv<>v<<<<v<^v>^<^^>>>^<v<v\n><>vv>v^v^<>><>>>><^^>vv>v<^^^>>v^v^<^^>v^^>v^<^v>v<>>v^v^<v>v^^<^^vv<\n<<v<^>>^^^^>>>v^<>vvv^><v<<<>^^^vv^<vvv>^>v<^^^^v<>^>vvvv><>>v^<<^^^^^\n^><^><>>><>^^<<^^v>>><^<v>^<vv>>v>>>^v><>^v><<<<v>>v<v<v>vvv>^<><<>^><\n^>><>^v<><^vvv<^^<><v<<<<<><^v<<<><<<^^<v<^^^><^>>^<v^><<<^>>^v<v^v<v^\n>^>>^v>vv>^<<^v<>><<><<v<<v><>v<^vv<<<>^^v^>^^>>><<^v>>v^v><^^>>^<>vv^\n<><^^>^^^<><vvvvv^v<v<<>^v<v>v<<^><<><<><<<^^<<<^<<>><<><^^^>^^<>^>v<>\n^^>vv<^v^v<vv>^<><v<^v>^^^>>>^^vvv^>vvv<>>>^<^>>>>>^<<^v>^vvv<>^<><<v>\nv^^>>><<^^<>>^v^<v^vv<>v^<<>^<^v^v><^<<<><<^<v><v<>vv>>v><v^<vv<>v^<<^"
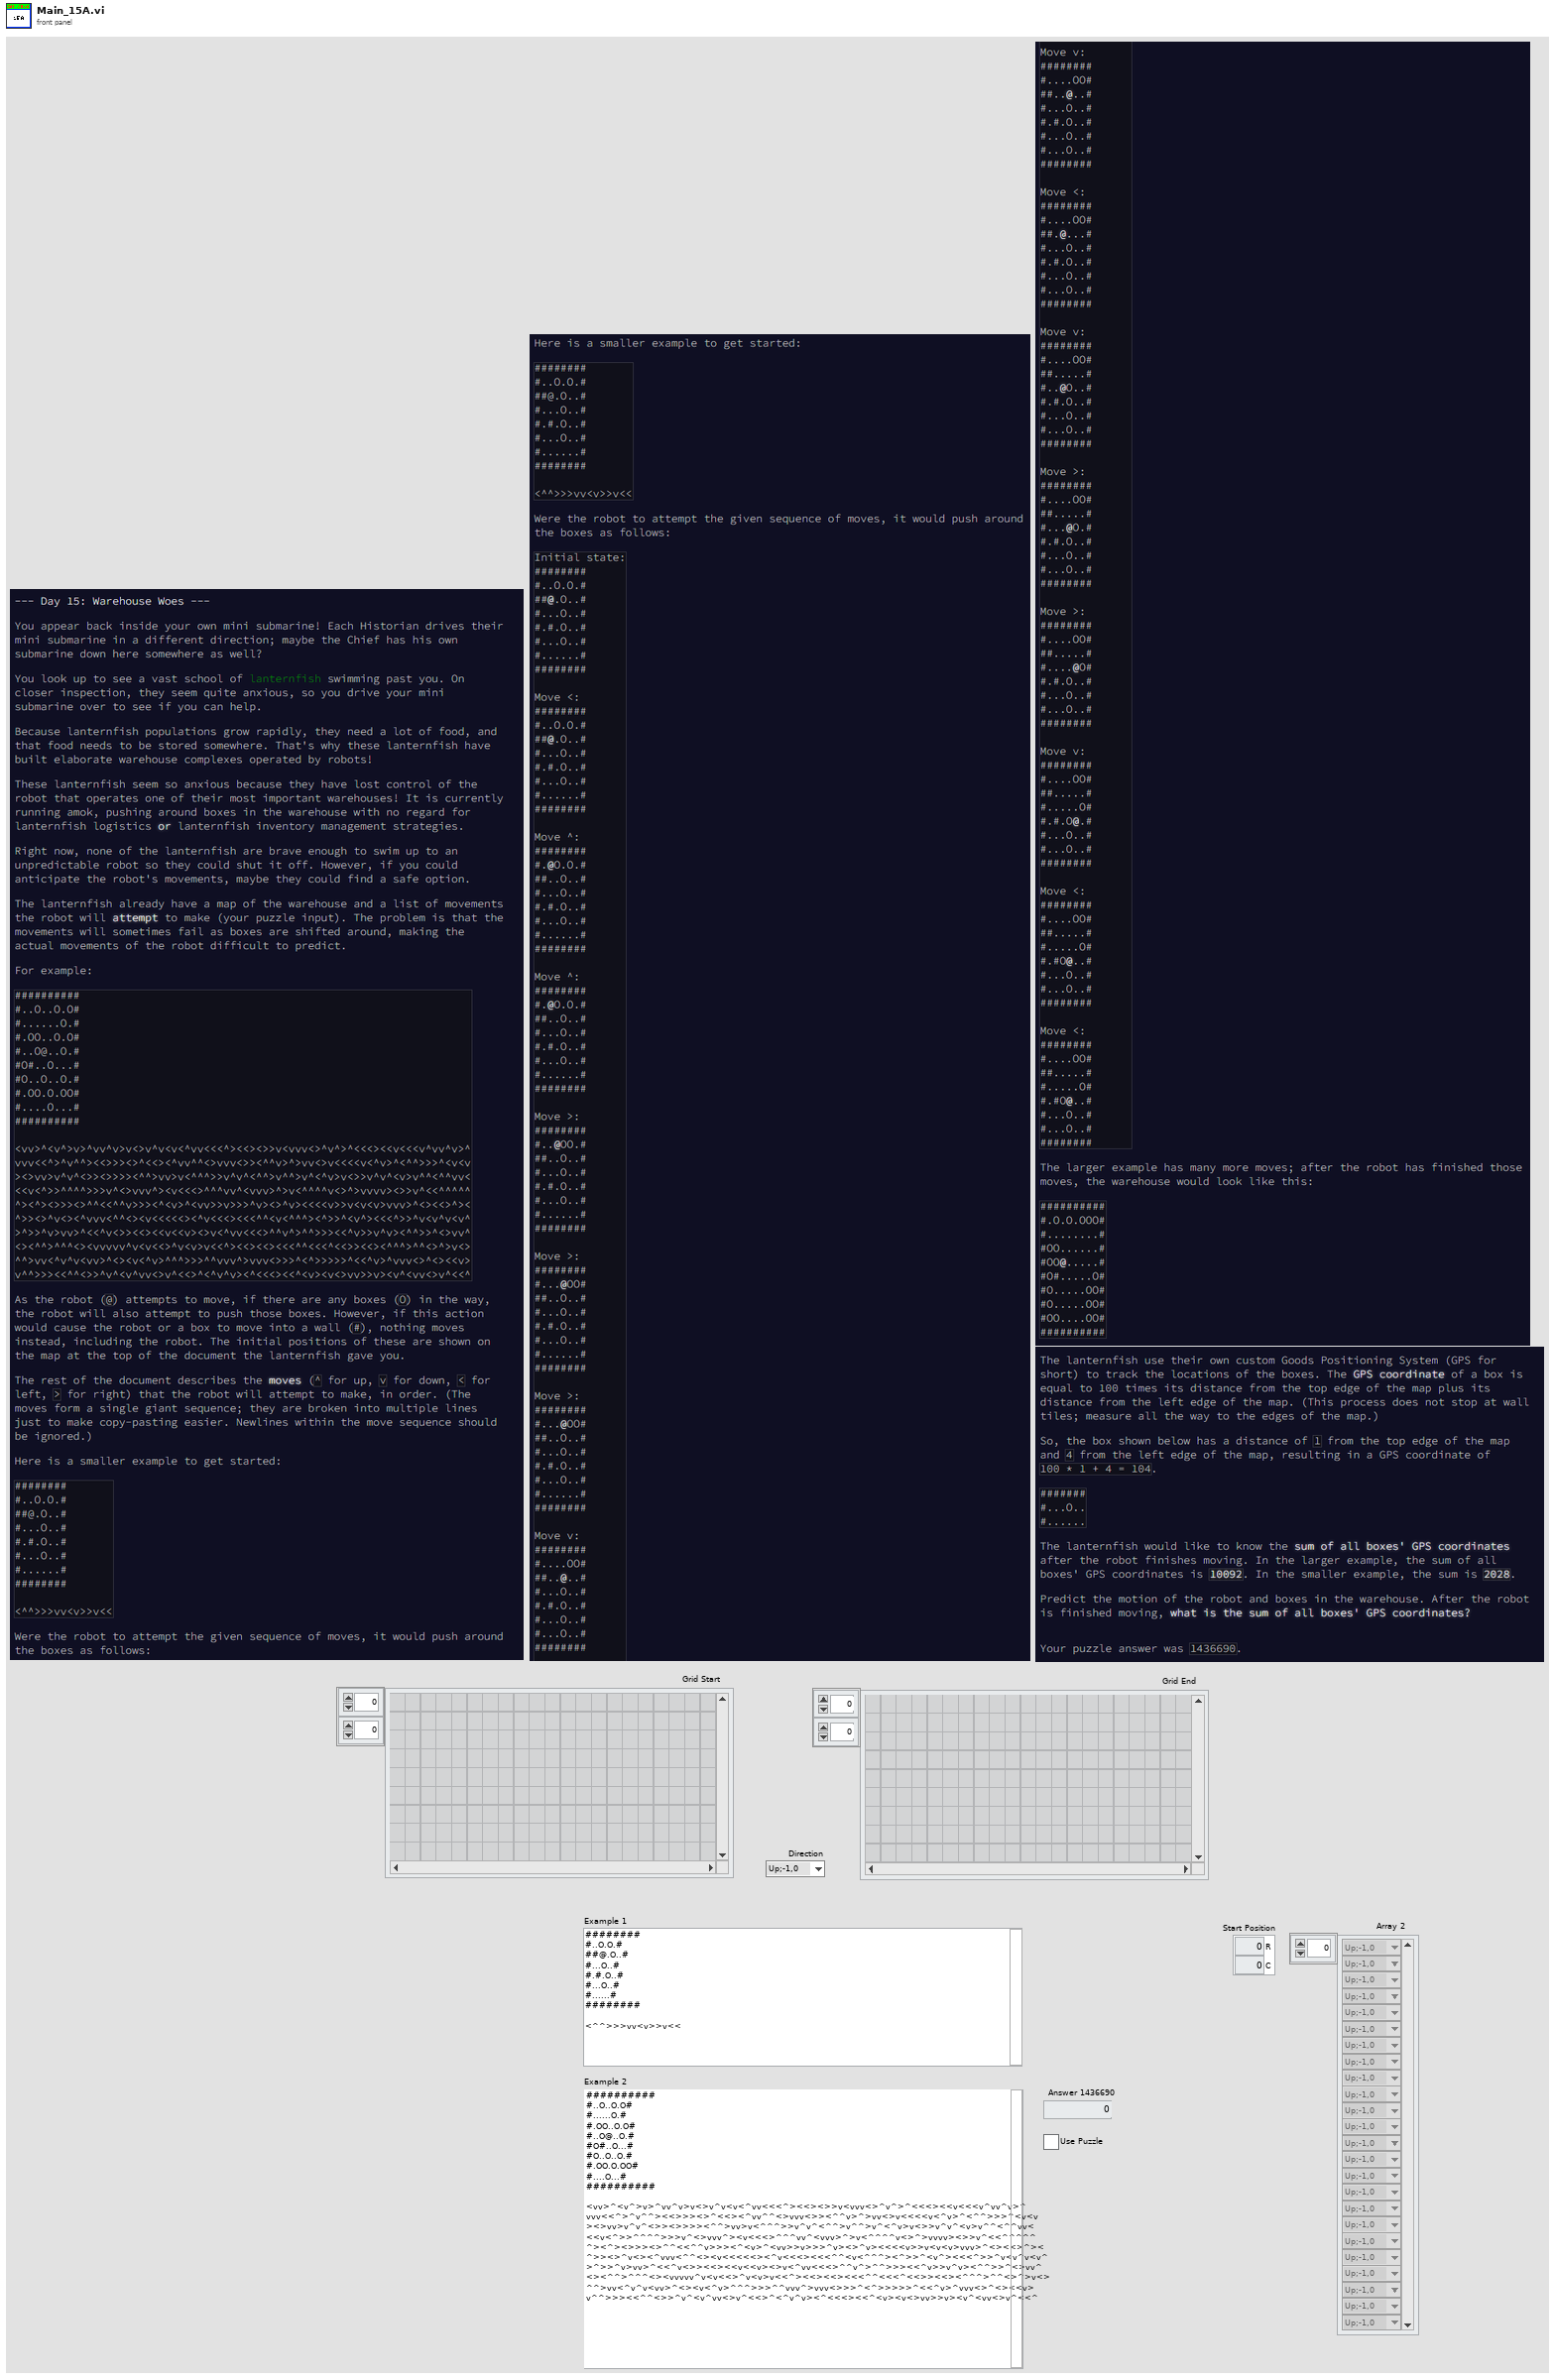
[diagram p1: front panel]
types:
  T1 = typedef "ENUM_4 Directions U-D-L-R.ctl" = enum16{"Up;-1,0", "Right;0,1", "Down;1,0", "Left;0,-1"}
  T2 = typedef "Cluster_Row-Column.ctl" = cluster{"R":i32, "C":i32}
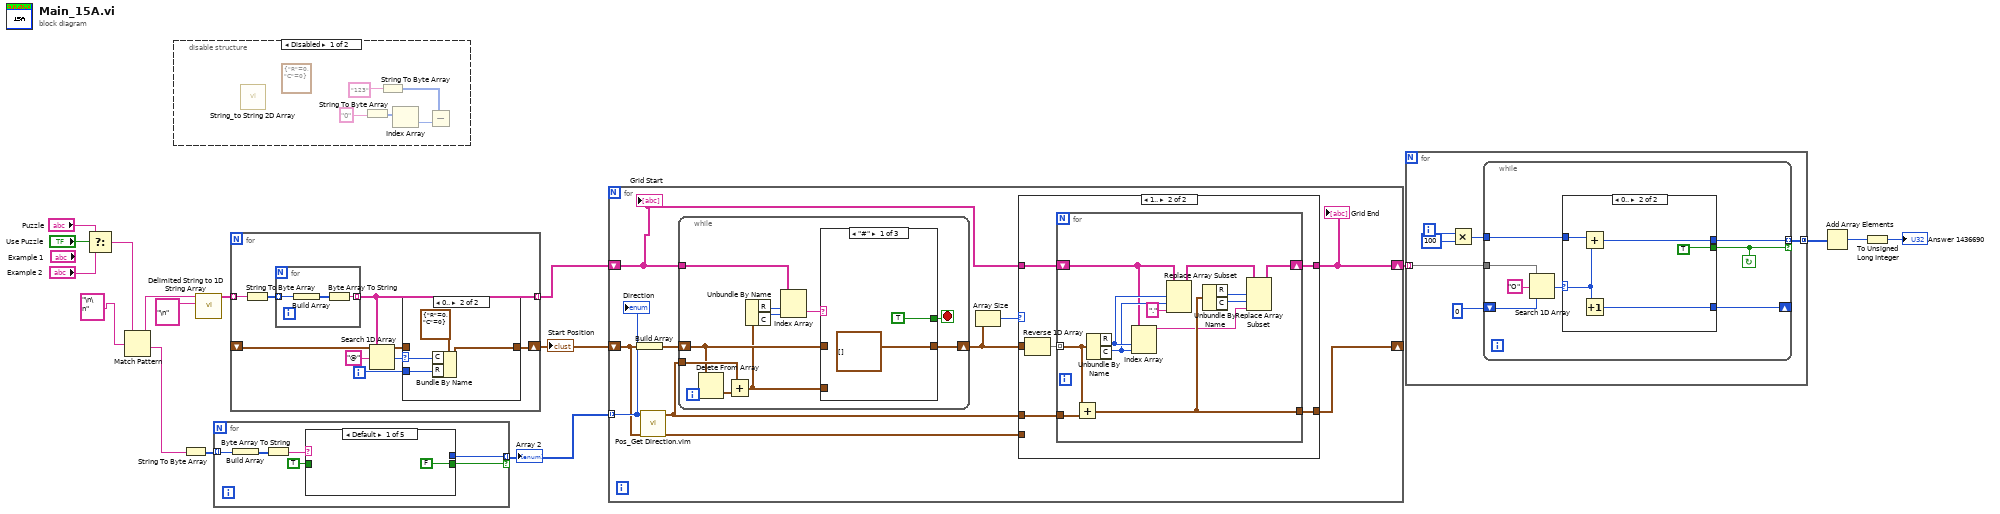
[diagram p0: block diagram]
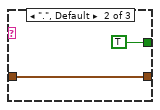
[diagram p4: hidden frame]
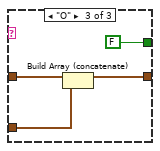
[diagram p5: hidden frame]
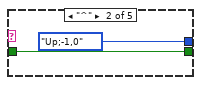
[diagram p6: hidden frame]
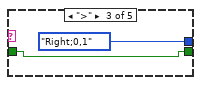
[diagram p7: hidden frame]
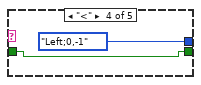
[diagram p8: hidden frame]
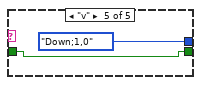
[diagram p9: hidden frame]
diagram:
  n1 = Select(t="Puzzle", s="Use Puzzle", f="Example 2") -> (s? t:f=w12:string)
  n2 = Match Pattern(string=w12, regular expression="\n\n" ("delimiter (Tab)")) -> (before substring=w11:string, after substring=w8:string)  [unwired: 1 in, 2 out]
  n3 = disable-structure shown="Disabled" {
    frame Disabled {
      (unwired) T2 {"R"=0, "C"=0} ("Position")
      n4 = call "String_to String 2D Array.vi"() -> ()  [unwired: 11 in, 1 out]
      n5 = String To Byte Array(string="0") -> (unsigned byte array=w20:u8[])
      n6 = String To Byte Array(string="123") -> (unsigned byte array=w18:u8[])
      n7 = Index Array(array=w20) -> (element=w19:u8)  [unwired: 1 in]
      n8 = Subtract(x=w18, y=w19) -> ()  [unwired: 1 out]
    }
    frame Enabled {
    }
  }
  n9 = String To Byte Array(string=w8) -> (unsigned byte array=w9:u8[])
  n10 = call <vilib>:"Delimited String to 1D String Array.vi"("delimiter"="\n" ("delimiter (Tab)"), "delimited string"=w11) -> ("string array"=w17:string[])  [unwired: 9 in]
  n11 = for {
    tunnel: w9 -> [w28] mode=indexing
    tunnel: [w25] -> w7 mode=indexing if=w23
    n12 = Build Array(w28) -> (w27:u8[])
    n13 = Byte Array To String(unsigned byte array=w27) -> (string=w26:string)
    n14 = case shown="Default" w26 {
      tunnel: [_ ENUM_4_Directions_U-D-L-R."Up;-1,0" ("Direction") ENUM_4_Directions_U-D-L-R."Right;0,1" ("Direction") ENUM_4_Directions_U-D-L-R."Left;0,-1" ("Direction") ENUM_4_Directions_U-D-L-R."Down;1,0" ("Direction")] -> w25
      tunnel: [FALSE w30 w32 w34 w36] -> w23
      tunnel: TRUE -> [_ w30 w32 w34 w36]
      frame Default {
      }
      frame "^" {
      }
      frame ">" {
      }
      frame "<" {
      }
      frame "v" {
      }
    }
  }
  "Array 2" <- w7
  n15 = for {
    tunnel: w17 -> [w44] mode=indexing
    shift-right: [w40] -> w5
    shift-left: _ -> [w39]
    tunnel: [w38] -> w6 mode=indexing
    i -> [w41]
    n16 = String To Byte Array(string=w44) -> (unsigned byte array=w45:u8[])
    n17 = for {
      tunnel: w45 -> [w53] mode=indexing
      tunnel: [w51] -> w38 mode=indexing
      n18 = Build Array(w53) -> (w52:u8[])
      n19 = Byte Array To String(unsigned byte array=w52) -> (string=w51:string)
    }
    n20 = Search 1D Array(1D array=w38, element="@") -> (index of element=w42:i32)  [unwired: 1 in]
    n21 = case shown="0.." w42 {
      selector: w42 -> [_ w49]
      tunnel: w41 -> [_ w48]
      tunnel: [w46 w47] -> w40
      tunnel: w39 -> [w46 _]
      frame ..-1 {
      }
      frame 0.. {
        n22 = Bundle By Name(cluster=T2 {"R"=0, "C"=0} ("Position"), "C"=w49, "R"=w48) -> (w47:T2)
      }
    }
  }
  "Start Position" <- w5
  n23 = for {
    tunnel: w7 -> [w62] mode=indexing
    shift-right: [w54] -> w2
    shift-left: w6 -> [w55]
    shift-right: [w59] -> _
    shift-left: w5 -> [w56]
    n24 = Build Array(w56) -> (w61:T2[])
    n25 = call "Pos_Get Direction.vim"("Direction"=w62) -> ("Position"=w60:T2)  [unwired: 10 in]
    n26 = while {
      tunnel: w60 -> [w91]
      shift-right: [w85] -> w58
      shift-left: w61 -> [w86]
      tunnel: w55 -> [w90]
      stop <- w84 stop-if-true
      n27 = Delete From Array(array=w86) -> (deleted portion=w92:T2)  [unwired: 2 in, 1 out]
      n28 = Add(x=w91, y=w92) -> (x+y=w83:T2)
      n29 = Unbundle By Name(w83) -> ("R"=w89:i32, "C"=w88:i32)
      n30 = Index Array(array=w90, index (row)=w89, index (col)=w88) -> (element=w87:string)
      n31 = case shown="\"#\"" w87 {
        tunnel: w86 -> [_ w95 w99]
        tunnel: [T2[] [] w95 w98] -> w85
        tunnel: [TRUE TRUE FALSE] -> w84
        tunnel: w83 -> [_ _ w97]
        frame "#" {
        }
        frame ".", Default {
        }
        frame "O" {
          n32 = Build Array (concatenate)(w99, w97) -> (w98:T2[])
        }
      }
    }
    n33 = Array Size(array=w58) -> (size(s)=w57:i32)
    n34 = case shown="1.." w57 {
      tunnel: w58 -> [_ w70]
      tunnel: w55 -> [w64 w69]
      tunnel: [w64 w68] -> w54
      tunnel: w60 -> [_ w66]
      tunnel: [w63 w65] -> w59
      tunnel: w56 -> [w63 _]
      frame ..0 {
      }
      frame 1.. {
        n35 = Reverse 1D Array(array=w70) -> (reversed array=w67:T2[])
        n36 = for {
          tunnel: w67 -> [w78] mode=indexing
          shift-right: [w77] -> w68
          shift-left: w69 -> [w72]
          tunnel: w66 -> [w79]
          tunnel: [w76] -> w65
          n37 = Add(x=w78, y=w79) -> (x+y=w76:T2)
          n38 = Unbundle By Name(w78) -> ("R"=w82:i32, "C"=w81:i32)
          n39 = Index Array(array=w72, index (row)=w82, index (col)=w81) -> (element=w73:string)
          n40 = Replace Array Subset(array=w72, new element="." ("new element/subarray"), index (row)=w82, index (col)=w81) -> (w71:string[][])
          n41 = Unbundle By Name(w76) -> ("R"=w75:i32, "C"=w74:i32)
          n42 = Replace Array Subset(array=w71, new element=w73, index (row)=w75, index (col)=w74) -> (w77:string[][])
        }
      }
    }
    "Grid End" <- w54
    "Grid Start" <- w55
    "Direction" <- w62
  }
  n43 = for {
    tunnel: w2 -> [w104] mode=indexing
    tunnel: [w101] -> w4 mode=concatenating
    i -> [w106]
    n44 = Multiply(x=w106, y=100) -> (x*y=w102:i32)
    n45 = while {
      tunnel: w104 -> [w114]
      shift-right: [w107] -> _
      shift-left: 0 -> [w111]
      tunnel: w102 -> [w110]
      tunnel: [w109] -> w101 mode=indexing if=w108
      stop <- w108 continue-if-true
      n46 = Search 1D Array(1D array=w114, element="O", start index (0)=w111) -> (index of element=w112:i32)
      n47 = case shown="0.." w112 {
        selector: w112 -> [_ w115]
        tunnel: w110 -> [_ w119]
        tunnel: [_ w118] -> w109
        tunnel: [_ TRUE] -> w108
        tunnel: [_ w116] -> w107
        frame ..-1 {
        }
        frame 0.. {
          n48 = Add(x=w119, y=w115) -> (x+y=w118:i32)
          n49 = Increment(x=w115) -> (x+1=w116:i32)
        }
      }
    }
  }
  n50 = Add Array Elements(numeric array=w4) -> (sum=w3:i32)
  n51 = To Unsigned Long Integer(number=w3) -> (unsigned 32bit integer=→"Answer 1436690":u32)
